vi "CRYIs Display Step.vi"(11 "pVIF_Out":refnum<vi>) -> (3 "Is Display Step?":bool)   [LabVIEW 2013]
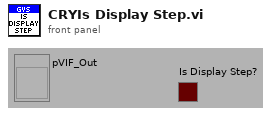
[diagram p1: front panel]
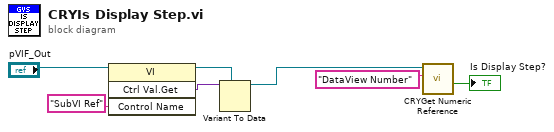
[diagram p0: block diagram]
diagram:
  n1 = invoke class="VI" method="Ctrl Val.Get"(reference="pVIF_Out", "Control Name"="SubVI Ref") -> (reference out=w4:refnum<vi>, "Get Control Value Variant"=w5:variant)  [unwired: 2 in, 2 out]
  n2 = Variant To Data(type=w4, Variant=w5) -> (data=w2:refnum<vi>)  [unwired: 1 in, 1 out]
  n3 = call "CRYGet Numeric Reference.vi"("Label Name"="DataView Number", "VI Refnum"=w2) -> ("Boolean"=→"Is Display Step?":bool)  [unwired: 9 out]
